vi "JSON Tree View Recursive.vi"(7 "error in (no error)":errorcluster, 8 "Item Indent In":i32, 9 "JSON Tree Expanded In":T1[](array[typedef]), 10 "JSON Tree":variant) -> (0 "error out":errorcluster, 2 "JSON Tree Expanded Out":T1[](array[typedef]))   [LabVIEW 2011, in "i3-json.lvlib"]
doc: "Use this template to build a VI to use as a subVI."
uses:
  i3-json.lvlib
  JSON Types/JSON Type.ctl
  Tree Nodes.ctl
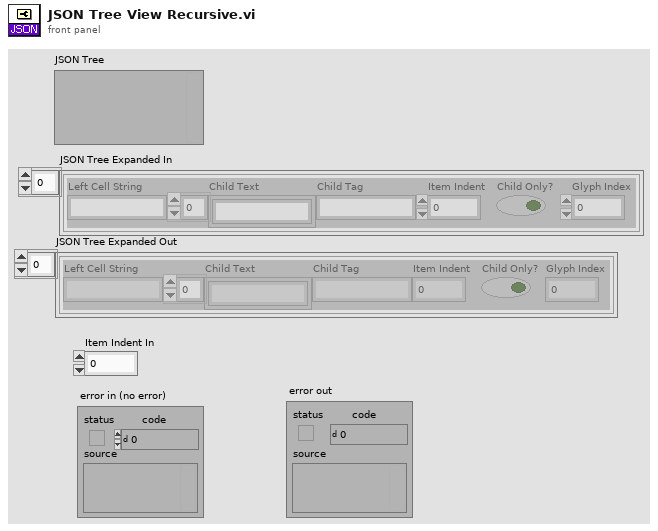
[diagram p1: front panel]
types:
  T1 = typedef "i3-json.lvlib/Tree Nodes.ctl" = cluster{"Left Cell String":string, "Child Text":string[], "Child Tag":string, "Item Indent":i32, "Child Only?":bool, "Glyph Index":i32}
  T2 = typedef "i3-json.lvlib/JSON Type.ctl" = enum8{"JSON Compatible", "JSON Array", "JSON Object", "JSON Null", "Double", "String", "Boolean", "Unknown", "Data JSON string"}
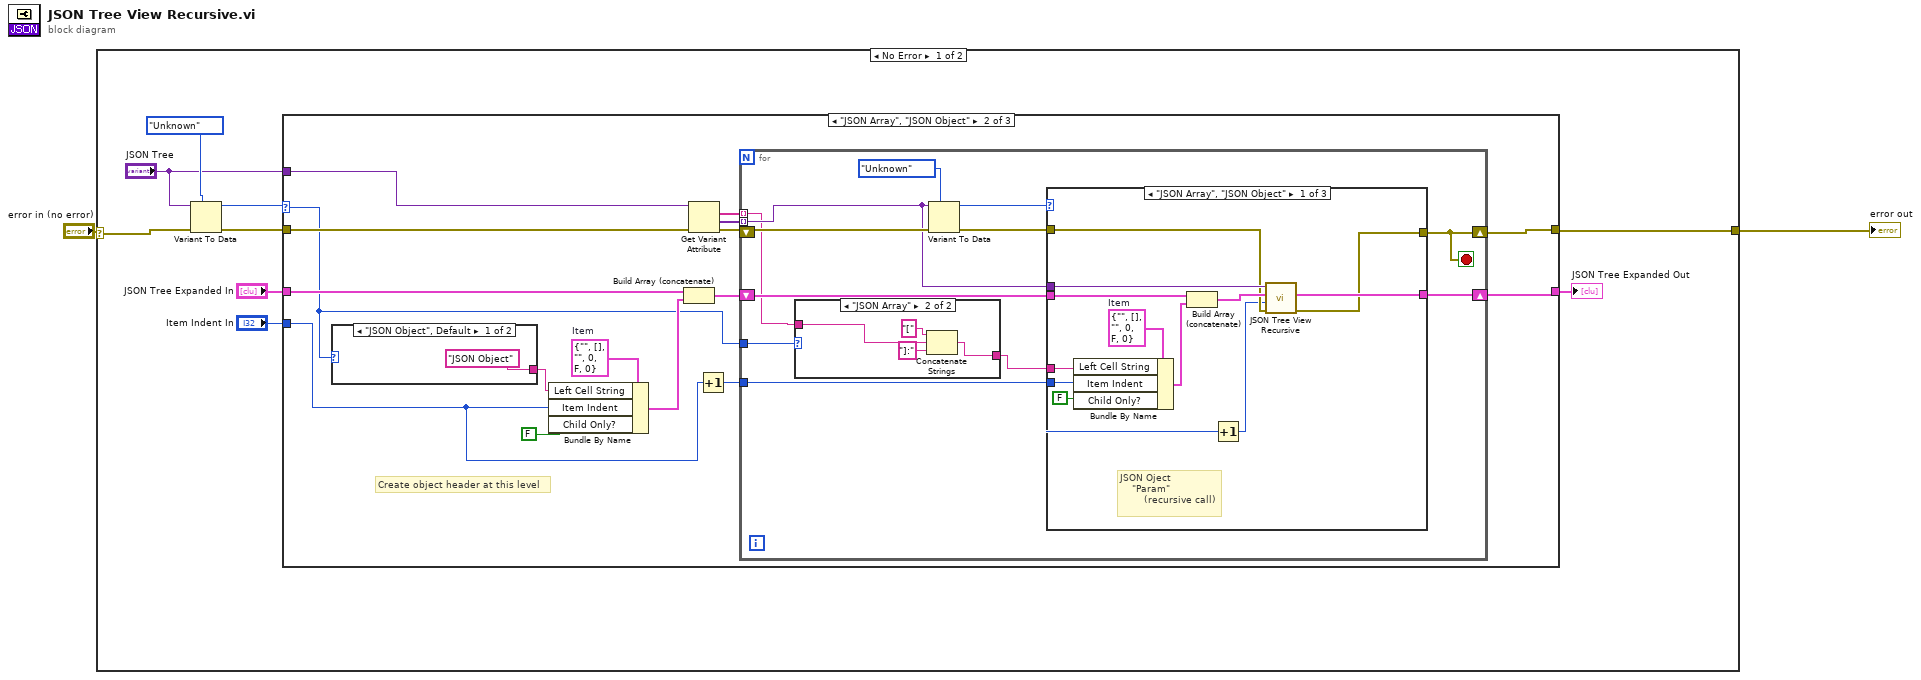
[diagram p0: block diagram]
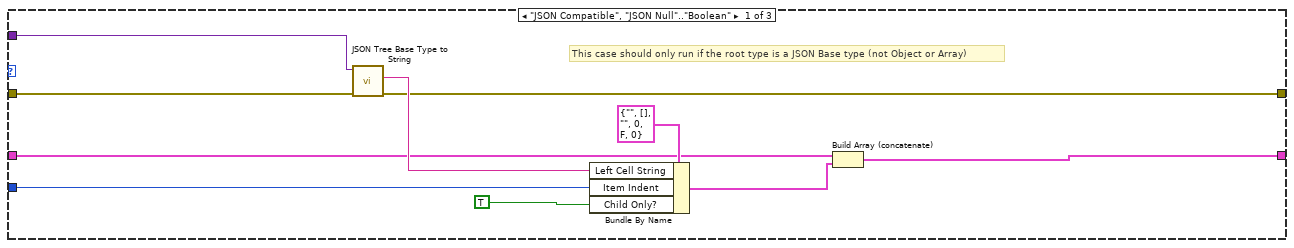
[diagram p2: hidden frame]
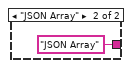
[diagram p3: hidden frame]
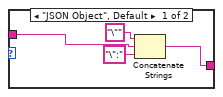
[diagram p4: hidden frame]
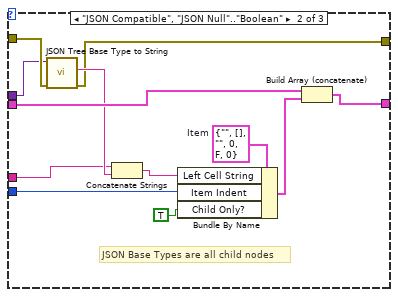
[diagram p5: hidden frame]
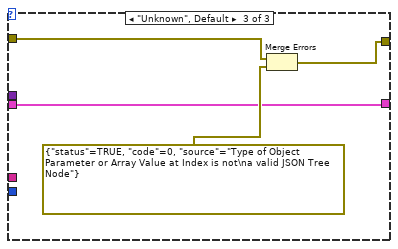
[diagram p6: hidden frame]
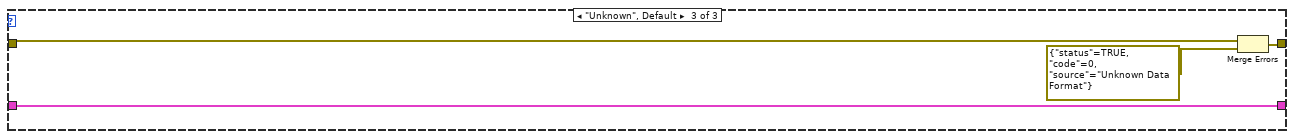
[diagram p7: hidden frame]
diagram:
  n1 = case shown="No Error" "error in (no error)" {
    selector: "error in (no error)" -> [w11 w92]
    tunnel: [w4 w92] -> w1
    frame No Error {
      n2 = Variant To Data(error in=w11, type=JSON_Type."Unknown" ("JSON Type"), Variant="JSON Tree") -> (data=w8:T2, error out=w10:errorcluster)
      n3 = case shown="\"JSON Array\", \"JSON Object\"" w8 {
        selector: w8 -> [_ w22 _]
        tunnel: w10 -> [w17 w37 w88]
        tunnel: "JSON Tree" -> [w15 w36 _]
        tunnel: "JSON Tree Expanded In" -> [w14 w33 w91]
        tunnel: "Item Indent In" -> [w19 w26 _]
        tunnel: [w16 w23 w90] -> w4
        tunnel: [w13 w24 w91] -> w3
        frame "JSON Compatible", "JSON Null".."Boolean" {
          # "This case should only run if the root type is a JSON Base type (not Object or Array)"
          n4 = call "JSON Tree Base Type to String.vi"("error in (no error)"=w17, "JSON Tree Base Type"=w15) -> ("error out"=w16:errorcluster, "JSON Tree Base Type String"=w18:string)  [unwired: 8 in]
          n5 = Bundle By Name(cluster=T1 {"Left Cell String"="", "Child Text"=[], "Child Tag"="", "Item Indent"=0, "Child Only?"=FALSE, "Glyph Index"=0} ("Item"), "Left Cell String"=w18, "Item Indent"=w19, "Child Only?"=TRUE) -> (w12:T1)
          n6 = Build Array (concatenate)(w14, w12) -> (w13:T1[])
        }
        frame "JSON Array", "JSON Object" {
          w31 = T1 {"Left Cell String"="", "Child Text"=[], "Child Tag"="", "Item Indent"=0, "Child Only?"=FALSE, "Glyph Index"=0}  # Item
          # "Create object header at this level"
          n7 = case shown="\"JSON Object\", Default" w22 {
            tunnel: ["JSON Object" "JSON Array"] -> w30
            frame "JSON Object", Default {
            }
            frame "JSON Array" {
            }
          }
          n8 = Bundle By Name(cluster=w31, "Left Cell String"=w30, "Item Indent"=w26, "Child Only?"=FALSE) -> (w28:T1)
          n9 = Build Array (concatenate)(w33, w28) -> (w32:T1[])
          n10 = Get Variant Attribute(Variant=w36, error in=w37) -> (names=w35:string[], values=w34:variant[], error out=w27:errorcluster)  [unwired: 2 in, 1 out]
          n11 = Increment(x=w26) -> (x+1=w25:i32)
          n12 = for {
            tunnel: w35 -> [w42] mode=indexing
            tunnel: w34 -> [w45] mode=indexing
            tunnel: w25 -> [w46]
            shift-right: [w44] -> w24
            shift-left: w32 -> [w47]
            tunnel: w22 -> [w40]
            shift-right: [w43] -> w23
            shift-left: w27 -> [w51]
            stop <- w43 stop-if-true
            n13 = case shown="\"JSON Array\"" w40 {
              tunnel: [w52 w56] -> w41
              tunnel: w42 -> [w54 w57]
              frame "JSON Object", Default {
                n14 = Concatenate Strings("\"" ("string"), w54, "\":" ("string")) -> (w52:string)
              }
              frame "JSON Array" {
                n15 = Concatenate Strings("[" ("string"), w57, "]:" ("string")) -> (w56:string)
              }
            }
            n16 = Variant To Data(error in=w51, type=JSON_Type."Unknown" ("JSON Type"), Variant=w45) -> (data=w48:T2, error out=w49:errorcluster)
            n17 = case shown="\"JSON Array\", \"JSON Object\"" w48 {
              tunnel: w49 -> [w65 w81 w86]
              tunnel: w41 -> [w60 w72 _]
              tunnel: w47 -> [w70 w79 w84]
              tunnel: w46 -> [w62 w77 _]
              tunnel: w45 -> [w66 w80 _]
              tunnel: [w64 w73 w84] -> w44
              tunnel: [w63 w74 w87] -> w43
              frame "JSON Array", "JSON Object" {
                w71 = T1 {"Left Cell String"="", "Child Text"=[], "Child Tag"="", "Item Indent"=0, "Child Only?"=FALSE, "Glyph Index"=0}  # Item
                # "JSON Oject\n    \"Param\"\n        (recursive call)"
                n18 = Bundle By Name(cluster=w71, "Left Cell String"=w60, "Item Indent"=w62, "Child Only?"=FALSE) -> (w68:T1)
                n19 = Build Array (concatenate)(w70, w68) -> (w67:T1[])
                n20 = Increment(x=w62) -> (x+1=w61:i32)
                n21 = call "JSON Tree View Recursive.vi"("error in (no error)"=w65, "Item Indent In"=w61, "JSON Tree Expanded In"=w67, "JSON Tree"=w66) -> ("error out"=w63:errorcluster, "JSON Tree Expanded Out"=w64:T1[])  [unwired: 5 in]
              }
              frame "JSON Compatible", "JSON Null".."Boolean" {
                w83 = T1 {"Left Cell String"="", "Child Text"=[], "Child Tag"="", "Item Indent"=0, "Child Only?"=FALSE, "Glyph Index"=0}  # Item
                # "JSON Base Types are all child nodes"
                n22 = call "JSON Tree Base Type to String.vi"("error in (no error)"=w81, "JSON Tree Base Type"=w80) -> ("error out"=w74:errorcluster, "JSON Tree Base Type String"=w76:string)  [unwired: 8 in]
                n23 = Concatenate Strings(w72, w76) -> (w75:string)
                n24 = Bundle By Name(cluster=w83, "Left Cell String"=w75, "Item Indent"=w77, "Child Only?"=TRUE) -> (w82:T1)
                n25 = Build Array (concatenate)(w79, w82) -> (w73:T1[])
              }
              frame "Unknown", Default {
                n26 = Merge Errors(w86, errorcluster {"status"=TRUE, "code"=0, "source"="Type of Object Parameter or Array Value at Index is not\na valid JSON Tree Node"} ("error out")) -> (w87:errorcluster)
              }
            }
          }
        }
        frame "Unknown", Default {
          n27 = Merge Errors(w88, errorcluster {"status"=TRUE, "code"=0, "source"="Unknown Data Format"} ("error in")) -> (w90:errorcluster)
        }
      }
      "JSON Tree Expanded Out" <- w3
    }
    frame Error {
    }
  }
  "error out" <- w1
